vi "exit.vi"(8 "error in (no error)":errorcluster, 10 "CommandID":i32, 11 "ContextThisComponent in":refnum<class "ContextThisComponent.lvclass">) -> (0 "error out":errorcluster, 3 "ContextThisComponent out":refnum<class "ContextThisComponent.lvclass">)   [LabVIEW 2016, in "ContextThisComponent.lvclass"]
uses:
  ContextThisComponent.lvclass
  ContextThisComponent.lvclass/ContextThisComponent.ctl
  IStateFactory/IStateFactory.lvclass
  IModel/IModel.lvclass
  State/State.lvclass
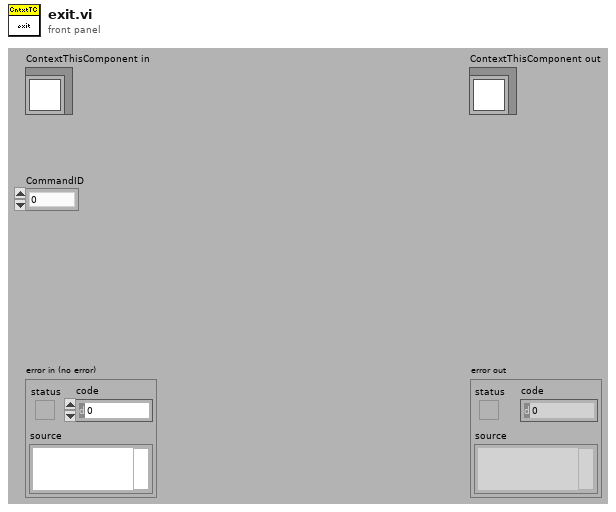
[diagram p1: front panel]
types:
  T1 = typedef "EXATypedefs.lvlib/StateValue.ctl" = enum16{"DisabledState", "EnabledState", "FaultState", "OffState", "StandbyState"}
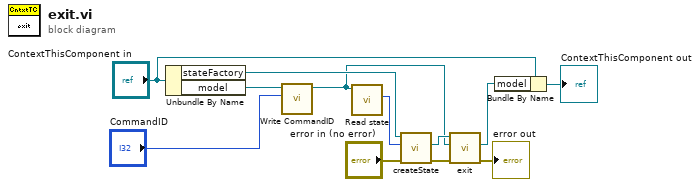
[diagram p0: block diagram]
diagram:
  n1 = Unbundle By Name("ContextThisComponent in") -> ("stateFactory"=w6:refnum<class "IStateFactory.lvclass">, "model"=w2:refnum<class "IModel.lvclass">)
  n2 = call-dynamic "Write CommandID.vi"("CommandID"="CommandID", "IModel in"=w2) -> ("IModel out"=w3:refnum<class "IModel.lvclass">)  [unwired: 8 in, 1 out]
  n3 = call-dynamic "Read state.vi"("IModel in"=w3) -> ("StateValue"=w4:T1)  [unwired: 9 in, 1 out]
  n4 = call-dynamic "createState.vi"("error in (no error)"="error in (no error)", "stateValue"=w4, "IStateFactory in"=w6) -> ("error out"=w5:errorcluster, "state"=w8:refnum<class "State.lvclass">)  [unwired: 6 in, 1 out]
  n5 = call-dynamic "exit.vi"("error in (no error)"=w5, "model in"=w3, "State in"=w8) -> ("error out"=→"error out":errorcluster, "model out"=w7:refnum<class "IModel.lvclass">)  [unwired: 6 in, 1 out]
  n6 = Bundle By Name(cluster="ContextThisComponent in", "model"=w7) -> (→"ContextThisComponent out":refnum<class "ContextThisComponent.lvclass">)
